vi "Day 4.1 - Winning score.vi"(11 "input":string[](array[string])) -> (3 "ouptut part 1":u64)   [LabVIEW 2021]
panel:
  out "Card":i32
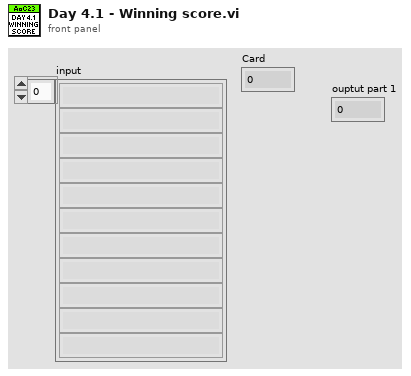
[diagram p1: front panel]
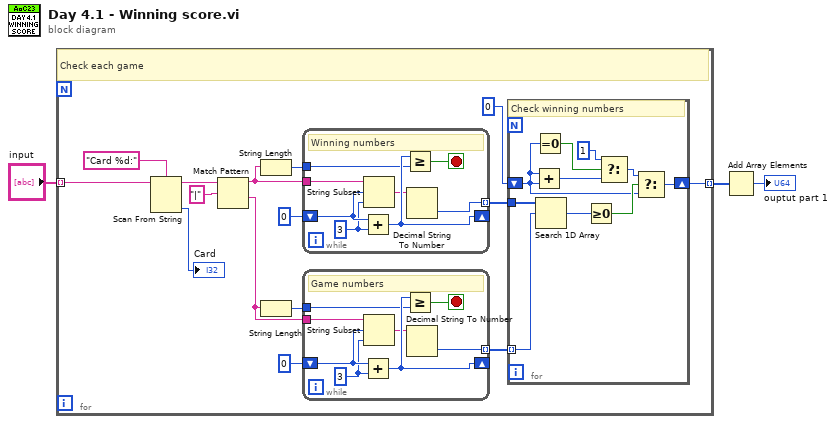
[diagram p0: block diagram]
diagram:
  n1 = for {
    tunnel: "input" -> [w18] mode=indexing
    tunnel: [w12] -> w1 mode=indexing
    # "Check each game"
    n2 = Scan From String(format string="Card %d:", input string=w18) -> (remaining string=w15:string, output 1=→"Card":i32)  [unwired: 3 in, 2 out]
    n3 = Match Pattern(string=w15, regular expression="|") -> (before substring=w10:string, after substring=w5:string)  [unwired: 1 in, 2 out]
    n4 = String Length(string=w10) -> (length=w9:i32)
    n5 = String Length(string=w5) -> (length=w7:i32)
    n6 = while {
      tunnel: w10 -> [w34]
      shift-right: [w30] -> _
      shift-left: 0 -> [w32]
      tunnel: w9 -> [w29]
      tunnel: [w27] -> w8 mode=indexing
      stop <- w33 stop-if-true
      w31 = 3 ("length (rest)")
      # "Winning numbers"
      n7 = Add(x=w32, y=w31) -> (x+y=w30:i32)
      n8 = String Subset(string=w34, offset (0)=w32, length (rest)=w31) -> (substring=w28:string)
      n9 = Greater Or Equal?(x=w30, y=w29) -> (x >= y?=w33:bool)
      n10 = Decimal String To Number(string=w28) -> (number=w27:i32)  [unwired: 2 in, 1 out]
    }
    n11 = while {
      tunnel: w5 -> [w26]
      shift-right: [w22] -> _
      shift-left: 0 -> [w24]
      tunnel: w7 -> [w21]
      tunnel: [w19] -> w4 mode=indexing
      stop <- w25 stop-if-true
      w23 = 3 ("length (rest)")
      # "Game numbers"
      n12 = Add(x=w24, y=w23) -> (x+y=w22:i32)
      n13 = String Subset(string=w26, offset (0)=w24, length (rest)=w23) -> (substring=w20:string)
      n14 = Greater Or Equal?(x=w22, y=w21) -> (x >= y?=w25:bool)
      n15 = Decimal String To Number(string=w20) -> (number=w19:i32)  [unwired: 2 in, 1 out]
    }
    n16 = for {
      tunnel: w4 -> [w43] mode=indexing
      tunnel: w8 -> [w44]
      shift-right: [w37] -> w12
      shift-left: 0 -> [w35]
      # "Check winning numbers"
      n17 = Add(x=w35, y=w35) -> (x+y=w36:i32)
      n18 = Equal To 0?(x=w35) -> (x = 0?=w40:bool)
      n19 = Search 1D Array(1D array=w44, element=w43) -> (index of element=w42:i32)  [unwired: 1 in]
      n20 = Greater Or Equal To 0?(x=w42) -> (x >= 0?=w41:bool)
      n21 = Select(t=1, s=w40, f=w36) -> (s? t:f=w38:i32)
      n22 = Select(t=w38, s=w41, f=w35) -> (s? t:f=w37:i32)
    }
  }
  n23 = Add Array Elements(numeric array=w1) -> (sum=→"ouptut part 1":i32)
